vi "Generate TCP Event Data.vi"(8 "error in (no error)":errorcluster, 9 "TCP Data":string, 10 "Connection ID":refnum<k5>, 11 "User Events.TCP RX":refnum<user-event>) -> (0 "error out":errorcluster)   [LabVIEW 2016, in "SLL Easy API via TCP.lvclass"]
uses:
  SLL Easy API via TCP.lvclass
  _Typedefs/TCP Event Data.ctl
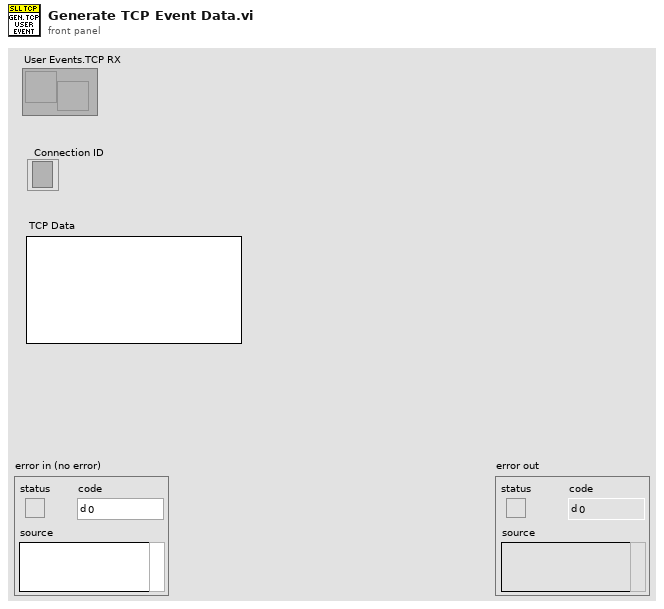
[diagram p1: front panel]
types:
  T1 = typedef "SLL Easy API via TCP.lvclass/TCP Event Data.ctl" = cluster{"Connection ID":refnum<k5>, "String":string}
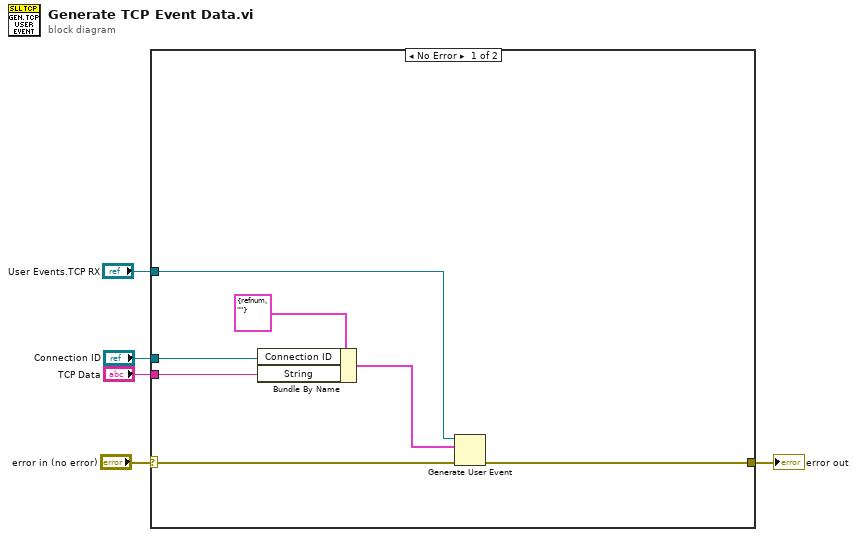
[diagram p0: block diagram]
diagram:
  n1 = case shown="No Error" "error in (no error)" {
    selector: "error in (no error)" -> [w12 w13]
    tunnel: "User Events.TCP RX" -> [w10 _]
    tunnel: [w11 w13] -> w3
    tunnel: "Connection ID" -> [w8 _]
    tunnel: "TCP Data" -> [w7 _]
    frame No Error {
      n2 = Bundle By Name(cluster=T1 {"Connection ID"=refnum, "String"=""} ("TCP Event Data"), "Connection ID"=w8, "String"=w7) -> (w6:T1)
      n3 = Generate User Event(user event=w10, event data cluster=w6, error in=w12) -> (error out=w11:errorcluster)  [unwired: 1 in, 1 out]
    }
    frame Error {
    }
  }
  "error out" <- w3
